vi "Wait for Configured Network on Address.vi"(9 "must be directly reachable?":bool, 10 "timeout in ms":i32=-1, 11 "address":string) -> (2 "resolved address":string, 3 "network status for remote host":T1)   [LabVIEW 2020, in "NI_WFCN.lvlib"]
doc: "Wait heuristically until the network configuration can contact the remote remote host. Generates no network traffic, but may execute system commands."
uses:
  <vilib>/net/WFCN/NI_WFCN.lvlib
  <vilib>/net/WFCN/Network Status.ctl
  <vilib>/net/WFCN/Addressing/IPv4 Network Address/IPv4 Network Address.lvclass/IPv4 Network Address.ctl
  <vilib>/net/WFCN/Addressing/Generic Network Address/Generic Network Address.lvclass/Generic Network Address.ctl
  <vilib>/net/WFCN/Addressing/Hostname Network Address/Hostname Network Address.lvclass/Hostname Network Address.ctl
  <vilib>/net/WFCN/Addressing/Hostname Network Address/Create from string.vi
  <vilib>/net/WFCN/Utility/Is IPv4 address.vi
  <vilib>/net/WFCN/Addressing/IPv4 Network Address/Create from U32.vi
  <vilib>/net/WFCN/Addressing/Generic Network Address/Create for unparsable.vi
  <vilib>/net/WFCN/Utility/Is hostname mDNS.vi
  <vilib>/dlg_ctls.llb/Space Constant.vi
  <vilib>/net/WFCN/Addressing/IPv4 Network Address/IPv4 Network Address.lvclass
  e:/builds/penguin/labview/branches/2020/dev/dist/vi.lib/net/WFCN/Addressing/Generic Network Address/Generic Network Address.lvclass
  <vilib>/net/WFCN/Addressing/Hostname Network Address/Hostname Network Address.lvclass
  <vilib>/net/WFCN/Addressing/mDNS Hostname Network Address/mDNS Hostname Network Address.lvclass
  e:/builds/penguin/labview/branches/2020/dev/dist/vi.lib/net/WFCN/Addressing/Hostname Network Address/Hostname Network Address.lvclass
  <vilib>/Utility/error.llb/Error Cluster From Error Code.vi
  <vilib>/UDC/API_Files/UDCCountUsage.vi
  <vilib>/net/WFCN/Addressing/Generic Network Address/Generic Network Address.lvclass
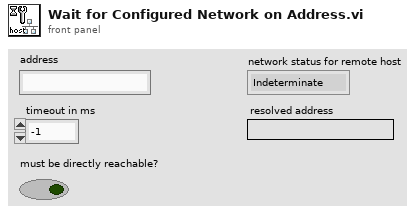
[diagram p1: front panel]
types:
  T1 = typedef "NI_WFCN.lvlib/Network Status.ctl" = enum16{"Indeterminate", "Configured", "Unconfigured"}
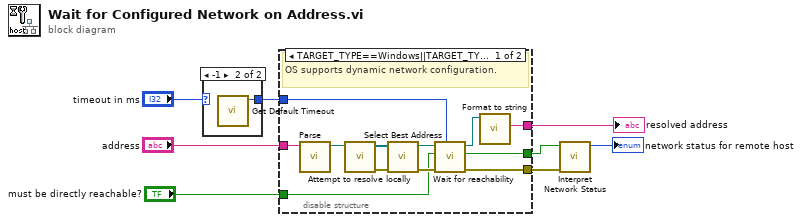
[diagram p0: block diagram]
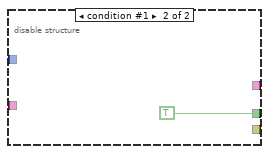
[diagram p2: hidden frame]
diagram:
  n1 = case shown="-1" "timeout in ms" {
    selector: "timeout in ms" -> [w9 _]
    tunnel: [w9 w10] -> w6
    frame 0, Default {
    }
    frame -1 {
      n2 = call <vilib>:"Get Default Timeout.vi"() -> ("default timeout (ms)"=w10:i32)  [unwired: 11 in]
    }
  }
  n3 = disable-structure shown="TARGET_TYPE==Windows||TARGET_TYPE==Mac||TARGET_TYPE==Unix||TARGET_TYPE==RT&&OS==Linux" {
    disable-tunnel: [w20 _] -> w2
    disable-tunnel: "address" -> [w22 _]
    disable-tunnel: w6 -> [w21 _]
    disable-tunnel: [w19 TRUE ("found?")] -> w5
    disable-tunnel: [w12 _] -> w3
    disable-tunnel: "must be directly reachable?" -> [w11 _]
    frame condition #0 (active) {
      # "OS supports dynamic network configuration."
      n4 = call <vilib>:"Parse.vi"("address string"=w22) -> ("address"=w18:refnum<class "Generic Network Address.lvclass">)  [unwired: 10 in]
      n5 = call-dynamic "Attempt to resolve locally.vi"("address"=w18) -> ("error out"=w17:errorcluster, "addresses out"=w15:refnum<class "Generic Network Address.lvclass">[])  [unwired: 9 in]
      n6 = call <vilib>:"Select Best Address.vi"("error in (no error)"=w17, "addresses"=w15) -> ("error out"=w16:errorcluster, "address"=w14:refnum<class "Generic Network Address.lvclass">)  [unwired: 7 in, 1 out]
      n7 = call-dynamic "Wait for reachability.vi"("timeout (ms)"=w21, "error in (no error)"=w16, "must be directly reachable?"=w11, "address"=w14) -> ("error out"=w20:errorcluster, "found?"=w19:bool, "address out"=w13:refnum<class "Generic Network Address.lvclass">)  [unwired: 5 in]
      n8 = call-dynamic "Format to string.vi"("address"=w13) -> ("address string"=w12:string)  [unwired: 8 in, 2 out]
    }
    frame condition #1 {
    }
  }
  "resolved address" <- w3
  n9 = call <vilib>:"Interpret Network Status.vi"("error in (no error)"=w2, "found?"=w5) -> ("network status for remote host"=→"network status for remote host":T1)  [unwired: 9 in]
